vi "Object type.vi"(4 "New version":string, 6 "App Name":string="My Application", 8 "error in":errorcluster, 9 "Build Object type":T1, 11 "Project Item Ref":refnum<vi>) -> (0 "error out":errorcluster)   [LabVIEW 2021, in "App-Builder Library.lvlib" / "Builder.lvclass"]
uses:
  Builder.lvclass
  Builder.lvclass/Builder.ctl
  <vilib>/regexp/Match Regular Expression.xnode
  Build object type.ctl
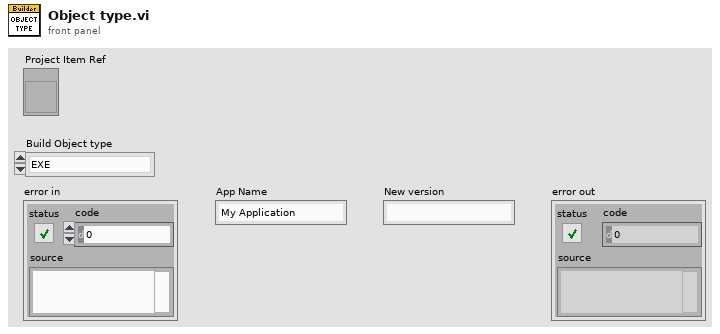
[diagram p1: front panel]
types:
  T1 = typedef "App-Builder Library.lvlib/Builder.lvclass/Build object type.ctl" = enum16{"EXE", "RT EXE", "Deployable Packed"}
  T2 = cluster{"Tag":enum16{"Bld_buildSpecDescription", "Bld_buildSpecName", "Bld_excludeLibraryItems", "Bld_excludePolymorphicVIs", "Bld_localDestDir", "Bld_modifyLibraryFile", "TgtF_autoIncrement", "TgtF_companyName", "TgtF_fileDescription", "TgtF_fileVersion.major", "TgtF_fileVersion.minor", "TgtF_fileVersion.patch", "TgtF_fileVersion.build", "TgtF_internalName", "TgtF_legalCopyright", "TgtF_productName", "TgtF_targetfileName"}, "Data":variant}
  T3 = cluster{"Tag":enum16{"Bld_buildSpecDescription", "Bld_buildSpecName", "Bld_excludeLibraryItems", "Bld_excludePolymorphicVIs", "Bld_localDestDir", "Bld_modifyLibraryFile", "TgtF_autoIncrement", "TgtF_companyName", "TgtF_fileDescription", "TgtF_fileVersion.major", "TgtF_fileVersion.minor", "TgtF_fileVersion.patch", "TgtF_fileVersion.build", "TgtF_internalName", "TgtF_legalCopyright", "TgtF_productName", "TgtF_targetfileName", "TgtF_packageName"}, "Data":variant}
  T4 = enum16{"Bld_buildSpecDescription", "Bld_buildSpecName", "Bld_excludeLibraryItems", "Bld_excludePolymorphicVIs", "Bld_localDestDir", "Bld_modifyLibraryFile", "TgtF_autoIncrement", "TgtF_companyName", "TgtF_fileDescription", "TgtF_fileVersion.major", "TgtF_fileVersion.minor", "TgtF_fileVersion.patch", "TgtF_fileVersion.build", "TgtF_internalName", "TgtF_legalCopyright", "TgtF_productName", "TgtF_targetfileName"}
  T5 = enum16{"Bld_buildSpecDescription", "Bld_buildSpecName", "Bld_excludeLibraryItems", "Bld_excludePolymorphicVIs", "Bld_localDestDir", "Bld_modifyLibraryFile", "TgtF_autoIncrement", "TgtF_companyName", "TgtF_fileDescription", "TgtF_fileVersion.major", "TgtF_fileVersion.minor", "TgtF_fileVersion.patch", "TgtF_fileVersion.build", "TgtF_internalName", "TgtF_legalCopyright", "TgtF_productName", "TgtF_targetfileName", "TgtF_packageName"}
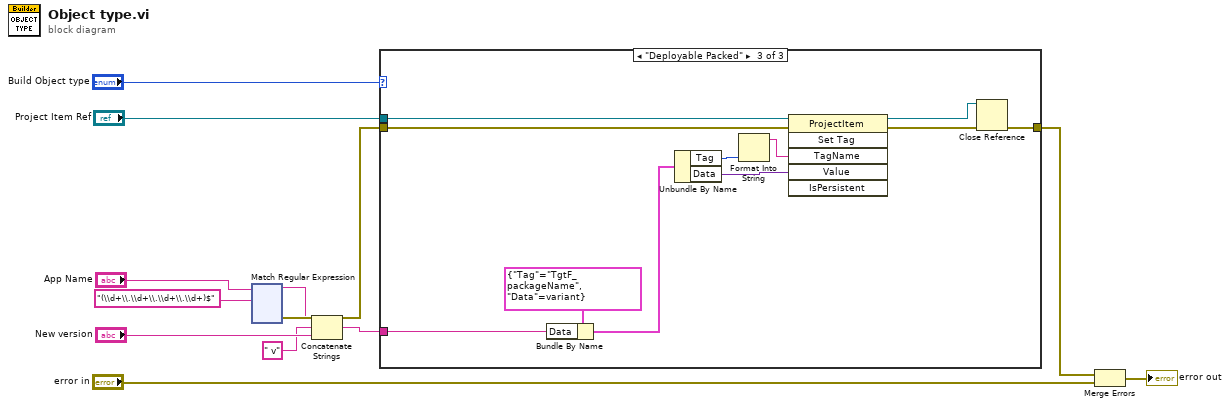
[diagram p0: block diagram]
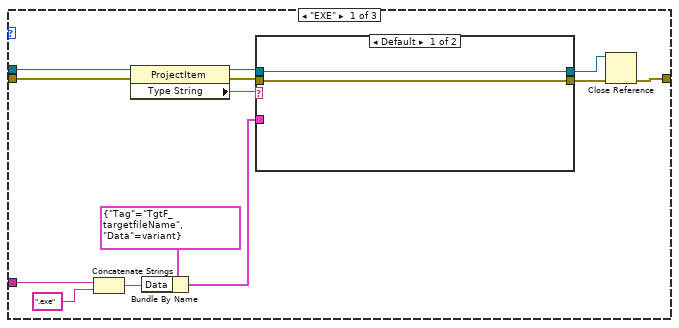
[diagram p2: hidden frame]
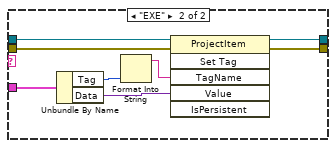
[diagram p3: hidden frame]
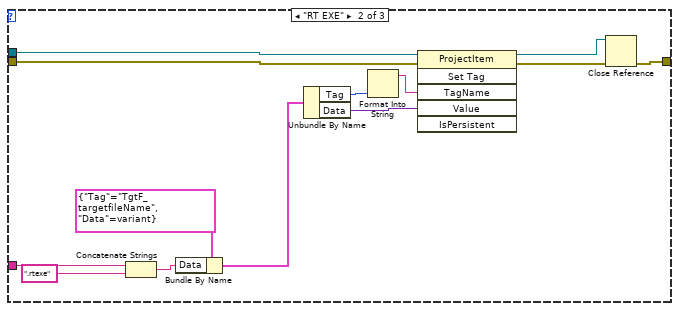
[diagram p4: hidden frame]
diagram:
  n1 = xnode "Match Regular Expression"("input string"="App Name", "regular expression"="(\\d+\\.\\d+\\.\\d+\\.\\d+)$") -> ("before match"=w2:string, "error out"=w8:errorcluster)  [unwired: 4 in, 3 out]
  n2 = Concatenate Strings(w2, " v" ("string"), "New version") -> (w11:string)
  n3 = case shown="\"Deployable Packed\"" "Build Object type" {
    tunnel: w11 -> [w15 w48 w59]
    tunnel: [w23 w45 w56] -> w10
    tunnel: "Project Item Ref" -> [w22 w44 w55]
    tunnel: w8 -> [w21 w43 w54]
    frame "EXE" {
      n4 = Concatenate Strings(w15, ".exe" ("string")) -> (w14:string)
      n5 = property class="ProjectItem"(reference=w22, error in=w21) -> (reference out=w17:refnum<vi>, error out=w16:errorcluster, "Type String"=w18:string)
      n6 = Bundle By Name(cluster=T2 {"Tag"=enum."TgtF_targetfileName", "Data"=variant}, "Data"=w14) -> (w25:T2)
      n7 = case shown="Default" w18 {
        tunnel: w17 -> [w26 w35]
        tunnel: [w27 w32] -> w20
        tunnel: w16 -> [w27 w34]
        tunnel: w25 -> [_ w33]
        tunnel: [w26 w31] -> w19
        frame Default {
        }
        frame "EXE" {
          n8 = Unbundle By Name(w33) -> ("Tag"=w29:T4, "Data"=w30:variant)
          n9 = Format Into String(w29) -> (resulting string=w28:string)  [unwired: 3 in, 1 out]
          n10 = invoke class="ProjectItem" method="Set Tag"(reference=w35, error in=w34, "TagName"=w28, "Value"=w30) -> (reference out=w31:refnum<vi>, error out=w32:errorcluster)  [unwired: 2 in, 4 out]
        }
      }
      n11 = Close Reference(reference=w19, error in (no error)=w20) -> (error out=w23:errorcluster)
    }
    frame "RT EXE" {
      n12 = Concatenate Strings(w48, ".rtexe" ("string")) -> (w37:string)
      n13 = Bundle By Name(cluster=T2 {"Tag"=enum."TgtF_targetfileName", "Data"=variant}, "Data"=w37) -> (w47:T2)
      n14 = Unbundle By Name(w47) -> ("Tag"=w39:T4, "Data"=w40:variant)
      n15 = Format Into String(w39) -> (resulting string=w38:string)  [unwired: 3 in, 1 out]
      n16 = invoke class="ProjectItem" method="Set Tag"(reference=w44, error in=w43, "TagName"=w38, "Value"=w40) -> (reference out=w41:refnum<vi>, error out=w42:errorcluster)  [unwired: 2 in, 4 out]
      n17 = Close Reference(reference=w41, error in (no error)=w42) -> (error out=w45:errorcluster)
    }
    frame "Deployable Packed" {
      n18 = Bundle By Name(cluster=T3 {"Tag"=enum."TgtF_packageName", "Data"=variant}, "Data"=w59) -> (w58:T3)
      n19 = Unbundle By Name(w58) -> ("Tag"=w50:T5, "Data"=w51:variant)
      n20 = Format Into String(w50) -> (resulting string=w49:string)  [unwired: 3 in, 1 out]
      n21 = invoke class="ProjectItem" method="Set Tag"(reference=w55, error in=w54, "TagName"=w49, "Value"=w51) -> (reference out=w52:refnum<vi>, error out=w53:errorcluster)  [unwired: 2 in, 4 out]
      n22 = Close Reference(reference=w52, error in (no error)=w53) -> (error out=w56:errorcluster)
    }
  }
  n23 = Merge Errors(w10, "error in") -> (→"error out":errorcluster)
